vi "solar_write LogWrite.vi"(8 "error in (no error)":errorcluster, 10 "Message":string, 11 "solar in":refnum<class "solar.lvclass">) -> (0 "error out":errorcluster, 3 "solar out":refnum<class "solar.lvclass">)   [LabVIEW 2018, in "solar.lvclass"]
doc: "This write the message to the solar log file as 'INFO:...'"
uses:
  solar.lvclass
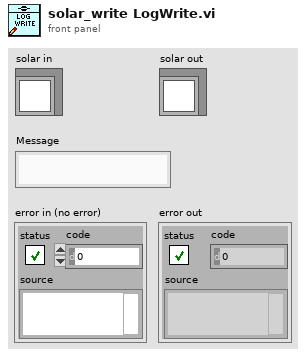
[diagram p1: front panel]
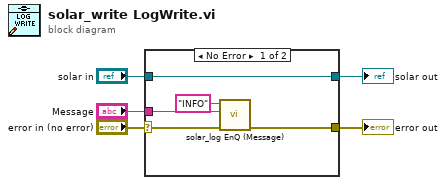
[diagram p0: block diagram]
diagram:
  n1 = case shown="No Error" "error in (no error)" {
    selector: "error in (no error)" -> [w9 w12]
    tunnel: "solar in" -> [w10 w11]
    tunnel: [w6 w12] -> w4
    tunnel: [w10 w11] -> w2
    tunnel: "Message" -> [w8 _]
    frame No Error {
      n2 = call "solar_log EnQ (Message).vi"("error in (no error)"=w9, "MSG"=w8, "Target"="INFO") -> ("error out"=w6:errorcluster)  [unwired: 8 in]
    }
    frame Error {
    }
  }
  "error out" <- w4
  "solar out" <- w2
